vi "Query Remote Trace Connection List Section.vi"(8 "error in (no error)":errorcluster, 11 "VISA resource name":refnum<visa-resource-name>) -> (0 "error out":errorcluster, 2 "Connection List":string, 3 "VISA resource name out":refnum<visa-resource-name>)   [LabVIEW 2020, in "Rohde&Schwarz CMXP Base.lvlib"]
doc: "Queries the contents of the connection list. There is one set of results per connection:\n\n{<ConnectionId>, <TestEnvironment>, <TimeStamp>, <VisaResource>, <ConnectionType>}conn 1, {...}conn 2, {...}conn 3, ...\n\nAttribute:\nRSCMXPBASE_ATTR_REMOTE_TRACE_CONNECTION_LIST_SECTION\n\nRemote-control command:\nFETCh:BASE:RTRace:CONNection:ROWS?"
uses:
  <instrlib>/Rohde&Schwarz CMXP Base/Rohde&Schwarz CMXP Base.lvlib
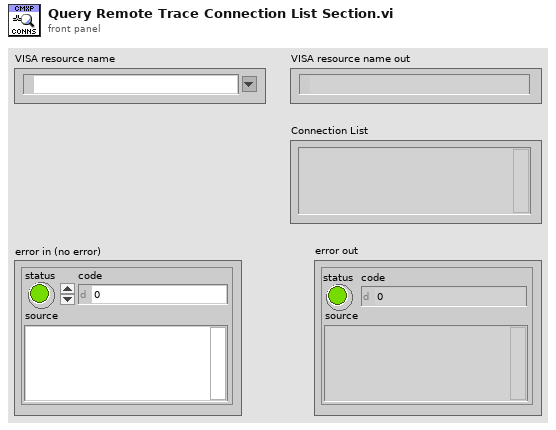
[diagram p1: front panel]
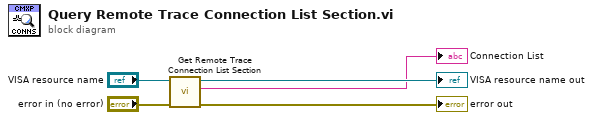
[diagram p0: block diagram]
diagram:
  n1 = call "Get Remote Trace Connection List Section"("error in (no error)"="error in (no error)", "instrument handle"="VISA resource name") -> ("error out"=→"error out":errorcluster, "Remote Trace Connection List Section"=→"Connection List":string, "instrument handle out"=→"VISA resource name out":refnum<visa-resource-name>)  [unwired: 7 in]
